vi "Make Vertical Location.vi"(6 "Side":T1=enum."right", 11 "Location":string) -> (0 "Vertical Location":T2)   [LabVIEW 2013]
uses:
  ROS/Code/SubVIs/BaxterSide.ctl
  Baxter Examples/Arm Globals.vi
  <vilib>/Utility/config.llb/Read Key (String).vi
  <vilib>/Utility/config.llb/NI_LVConfig.lvlib
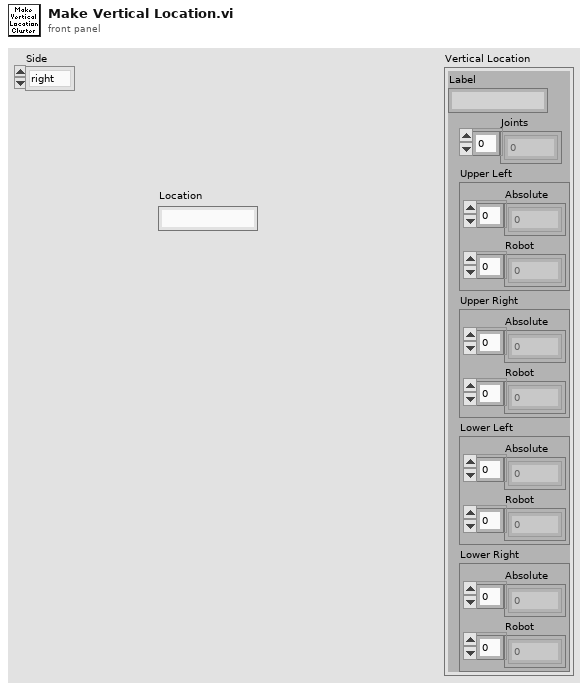
[diagram p1: front panel]
types:
  T1 = typedef "BaxterSide.ctl" = enum16{"left", "right"}
  T2 = cluster{"Label":string, "Joints":dbl[], "Upper Left":cluster{"Absolute":dbl[], "Robot":dbl[]}, "Upper Right":cluster{"Absolute":dbl[], "Robot":dbl[]}, "Lower Left":cluster{"Absolute":dbl[], "Robot":dbl[]}, "Lower Right":cluster{"Absolute":dbl[], "Robot":dbl[]}}
  T3 = typedef "NI_LVConfig.lvlib/Config Data RefNum.ctl" = refnum<k1>
  T4 = cluster{"Label":string, "Joints":dbl[], "Far Left":cluster{"Absolute":dbl[], "Robot":dbl[]}, "Far Right":cluster{"Absolute":dbl[], "Robot":dbl[]}, "Near Left":cluster{"Absolute":dbl[], "Robot":dbl[]}, "Near Right":cluster{"Absolute":dbl[], "Robot":dbl[]}}[]
  T5 = cluster{"Label":string, "Joints":dbl[], "Far Left":cluster{"Absolute":dbl[], "Robot":dbl[]}, "Far Right":cluster{"Absolute":dbl[], "Robot":dbl[]}, "Near Left":cluster{"Absolute":dbl[], "Robot":dbl[]}, "Near Right":cluster{"Absolute":dbl[], "Robot":dbl[]}}
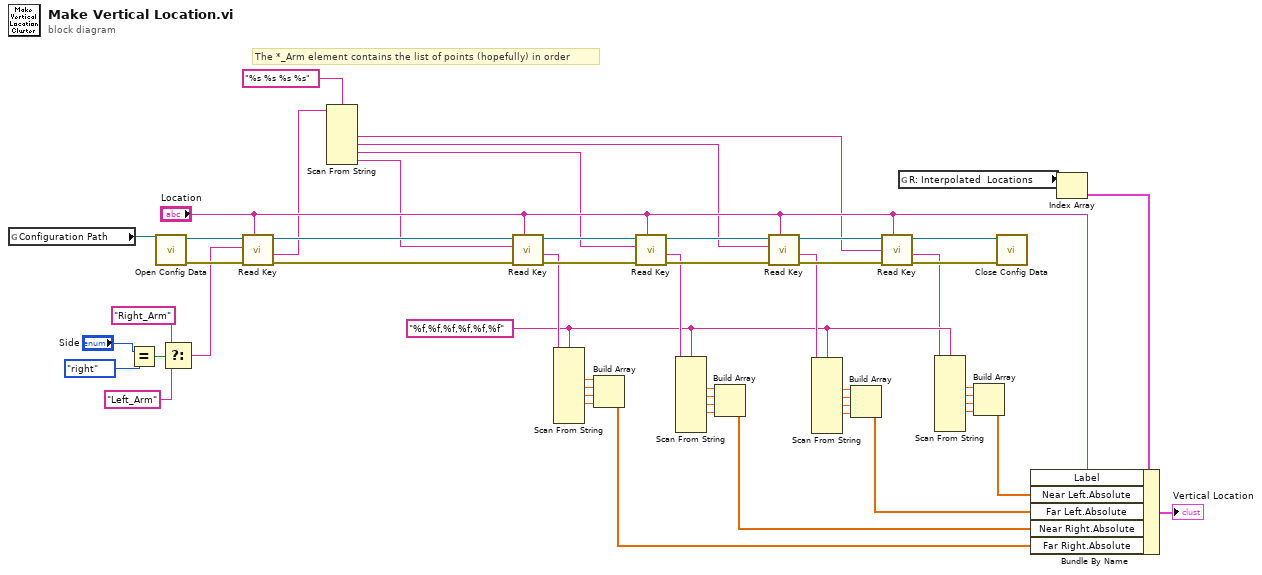
[diagram p0: block diagram]
diagram:
  w22 = "%f,%f,%f,%f,%f,%f" ("format string")
  # "The *_Arm element contains the list of points (hopefully) in order"
  n1 = global read "Arm Globals.vi" "Configuration Path"() -> (w54:path)
  n2 = Equal?(x="Side", y=BaxterSide."right" ("Side")) -> (x = y?=w11:bool)
  n3 = call <vilib>:"Open Config Data.vi"("configuration file path"=w54) -> ("error out"=w15:errorcluster, "refnum"=w17:T3)  [unwired: 8 in, 1 out]
  n4 = Select(t="Right_Arm", s=w11, f="Left_Arm") -> (s? t:f=w8:string)
  n5 = call-poly <vilib>:"Read Key.vi"("section"="Location", "error in (no error)"=w15, "key"=w8, "refnum"=w17) -> ("error out"=w14:errorcluster, "value"=w1:string, "refnum out"=w16:T3)  [unwired: 4 in, 1 out]
  n6 = Scan From String(format string="%s %s %s %s", input string=w1) -> (output 1=w3:string, output 2=w4:string, output 3=w5:string, output 4=w6:string)  [unwired: 6 in, 3 out]
  n7 = call-poly <vilib>:"Read Key.vi"("section"="Location", "error in (no error)"=w14, "key"=w6, "refnum"=w16) -> ("error out"=w53:errorcluster, "value"=w44:string, "refnum out"=w49:T3)  [unwired: 4 in, 1 out]
  n8 = Scan From String(format string=w22, input string=w44) -> (output 1=w42:dbl, output 2=w41:dbl, output 3=w40:dbl, output 4=w39:dbl)  [unwired: 10 in, 3 out]
  n9 = Build Array(w42, w41, w40, w39) -> (w33:dbl[])
  n10 = call-poly <vilib>:"Read Key.vi"("section"="Location", "error in (no error)"=w53, "key"=w5, "refnum"=w49) -> ("error out"=w52:errorcluster, "value"=w34:string, "refnum out"=w48:T3)  [unwired: 4 in, 1 out]
  n11 = Scan From String(format string=w22, input string=w34) -> (output 1=w38:dbl, output 2=w37:dbl, output 3=w36:dbl, output 4=w35:dbl)  [unwired: 10 in, 3 out]
  n12 = Build Array(w38, w37, w36, w35) -> (w32:dbl[])
  n13 = call-poly <vilib>:"Read Key.vi"("section"="Location", "error in (no error)"=w52, "key"=w4, "refnum"=w48) -> ("error out"=w51:errorcluster, "value"=w23:string, "refnum out"=w47:T3)  [unwired: 4 in, 1 out]
  n14 = Scan From String(format string=w22, input string=w23) -> (output 1=w31:dbl, output 2=w30:dbl, output 3=w29:dbl, output 4=w28:dbl)  [unwired: 10 in, 3 out]
  n15 = Build Array(w31, w30, w29, w28) -> (w19:dbl[])
  n16 = call-poly <vilib>:"Read Key.vi"("section"="Location", "error in (no error)"=w51, "key"=w3, "refnum"=w47) -> ("error out"=w50:errorcluster, "value"=w21:string, "refnum out"=w46:T3)  [unwired: 4 in, 1 out]
  n17 = global read "Arm Globals.vi" "R: Interpolated  Locations"() -> (w45:T4)
  n18 = Scan From String(format string=w22, input string=w21) -> (output 1=w27:dbl, output 2=w26:dbl, output 3=w25:dbl, output 4=w24:dbl)  [unwired: 10 in, 3 out]
  n19 = Build Array(w27, w26, w25, w24) -> (w20:dbl[])
  n20 = call <vilib>:"Close Config Data.vi"("error in (no error)"=w50, "refnum"=w46) -> ()  [unwired: 8 in, 2 out]
  n21 = Index Array(array=w45) -> (element=w43:T5)  [unwired: 1 in]
  n22 = Bundle By Name(cluster=w43, "Label"="Location", "Near Left.Absolute"=w20, "Far Left.Absolute"=w19, "Near Right.Absolute"=w32, "Far Right.Absolute"=w33) -> (→"Vertical Location":T5)
